vi "Page_Source_Supports_Configurable_VI.vi"(8 "error in (no error)":errorcluster, 11 "AB_WebService in":refnum<class "AB_WebService.lvclass">) -> (0 "error out":errorcluster, 2 "supports configurable VI":bool, 3 "AB_WebService out":refnum<class "AB_WebService.lvclass">)   [LabVIEW 2020, in "AB_WebService.lvclass"]
uses:
  <vilib>/AppBuilder/AB_Classes/WebService/AB_WebService.lvclass
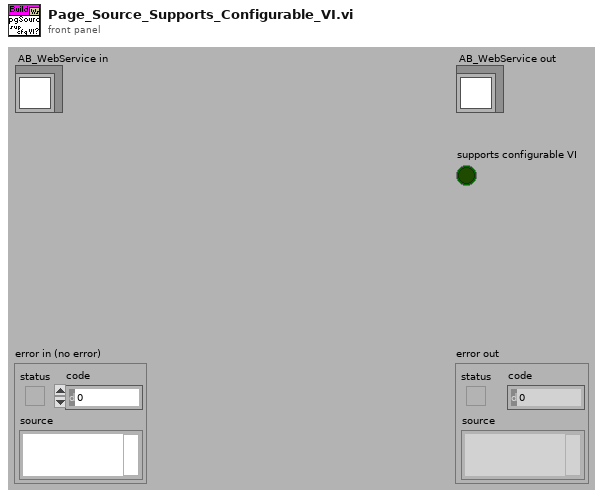
[diagram p1: front panel]
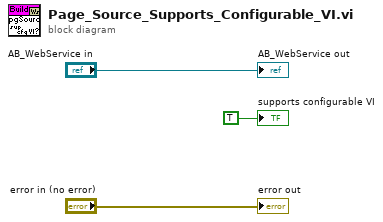
[diagram p0: block diagram]
diagram:
  "error out" <- "error in (no error)"
  "AB_WebService out" <- "AB_WebService in"
  "supports configurable VI" <- TRUE ("supports configurable VI")
